vi "StopWatch.vi"(5 "Action":enum16{"Start", "Stop", "Read", "Reset"}(ring)) -> (0 "Time paused":u32 format="%<%H:%M:%S>t", 1 "Status":enum16{"Resetted", "Paused", "Running"}(ring), 2 "Time elapsed":u32 format="%<%H:%M:%S>t", 3 "Time stopped":dbl format="%<%H:%M:%S>t", 4 "Time started":dbl format="%<%H:%M:%S>t")   [LabVIEW 2013]
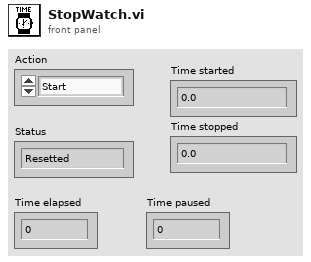
[diagram p1: front panel]
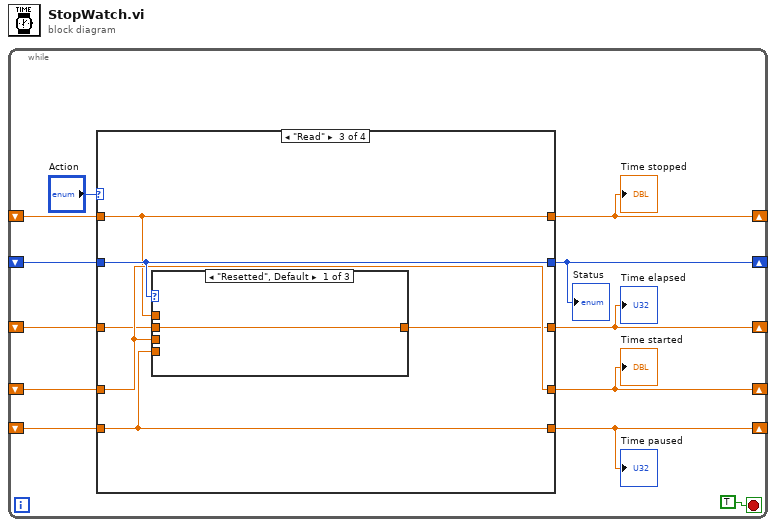
[diagram p0: block diagram]
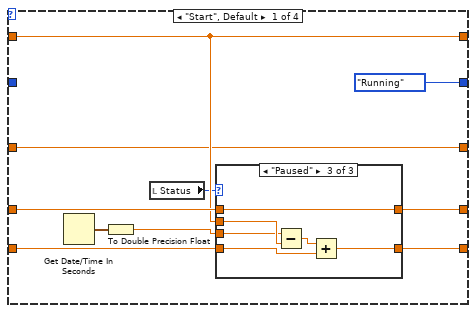
[diagram p2: hidden frame]
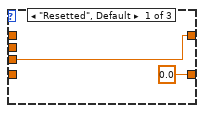
[diagram p3: hidden frame]
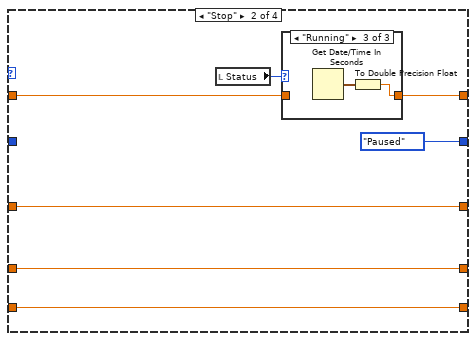
[diagram p5: hidden frame]
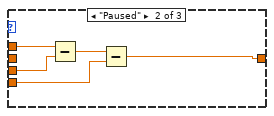
[diagram p8: hidden frame]
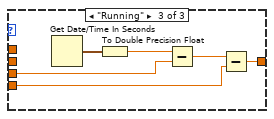
[diagram p9: hidden frame]
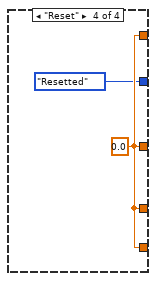
[diagram p10: hidden frame]
diagram:
  n1 = while {
    shift-right: [w3] -> _
    shift-left: _ -> [w9]
    shift-right: [w6] -> _
    shift-left: _ -> [w7]
    shift-right: [w1] -> _
    shift-left: _ -> [w11]
    shift-right: [w2] -> _
    shift-left: _ -> [w8]
    shift-right: [w5] -> _
    shift-left: _ -> [w4]
    stop <- TRUE stop-if-true
    n2 = case shown="\"Read\"" "Action" {
      tunnel: [enum16{"Resetted", "Paused", "Running"}."Running" ("Status") enum16{"Resetted", "Paused", "Running"}."Paused" ("Status") w49 enum16{"Resetted", "Paused", "Running"}."Resetted" ("Status")] -> w1
      tunnel: w11 -> [_ _ w49 _]
      tunnel: [w20 w38 w48 w63] -> w3
      tunnel: w9 -> [w17 w38 w48 _]
      tunnel: [w18 w39 w44 w63] -> w6
      tunnel: [w16 w33 w47 w63] -> w2
      tunnel: w8 -> [w16 w34 w47 _]
      tunnel: w7 -> [w19 w39 w44 _]
      tunnel: [w15 w37 w46 w63] -> w5
      tunnel: w4 -> [w15 w37 w45 _]
      frame "Start", Default {
        n3 = Get Date/Time In Seconds() -> (seconds since 1Jan1904=w22:timestamp)
        n4 = To Double Precision Float(number=w22) -> (double precision float=w21:dbl)
        n5 = local read "Status"() -> (w14:enum16{"Resetted", "Paused", "Running"})
        n6 = case shown="\"Paused\"" w14 {
          tunnel: w21 -> [w24 _ w31]
          tunnel: [w24 w26 w27] -> w20
          tunnel: w16 -> [_ _ w32]
          tunnel: w19 -> [_ w25 w30]
          tunnel: [0.0 w25 w28] -> w18
          tunnel: w17 -> [_ w26 w27]
          frame "Resetted", Default {
          }
          frame "Running" {
          }
          frame "Paused" {
            n7 = Subtract(x=w31, y=w32) -> (x-y=w29:dbl)
            n8 = Add(x=w29, y=w30) -> (x+y=w28:dbl)
          }
        }
      }
      frame "Stop" {
        n9 = local read "Status"() -> (w35:enum16{"Resetted", "Paused", "Running"})
        n10 = case shown="\"Running\"" w35 {
          tunnel: w34 -> [w40 w41 _]
          tunnel: [w40 w41 w42] -> w33
          frame "Resetted", Default {
          }
          frame "Paused" {
          }
          frame "Running" {
            n11 = Get Date/Time In Seconds() -> (seconds since 1Jan1904=w43:timestamp)
            n12 = To Double Precision Float(number=w43) -> (double precision float=w42:dbl)
          }
        }
      }
      frame "Read" {
        n13 = case shown="\"Resetted\", Default" w49 {
          tunnel: [w50 w53 w57] -> w46
          tunnel: w44 -> [_ w51 w56]
          tunnel: w48 -> [_ w55 w58]
          tunnel: w47 -> [_ w52 _]
          tunnel: w45 -> [w50 _ _]
          frame "Resetted", Default {
          }
          frame "Paused" {
            n14 = Subtract(x=w52, y=w55) -> (x-y=w54:dbl)
            n15 = Subtract(x=w54, y=w51) -> (x-y=w53:dbl)
          }
          frame "Running" {
            n16 = Get Date/Time In Seconds() -> (seconds since 1Jan1904=w61:timestamp)
            n17 = To Double Precision Float(number=w61) -> (double precision float=w60:dbl)
            n18 = Subtract(x=w60, y=w58) -> (x-y=w59:dbl)
            n19 = Subtract(x=w59, y=w56) -> (x-y=w57:dbl)
          }
        }
      }
      frame "Reset" {
        w63 = 0.0
      }
    }
    "Time paused" <- w6
    "Time elapsed" <- w5
    "Time started" <- w3
    "Time stopped" <- w2
    "Status" <- w1
  }
